vi "Stop Work.vi"(8 "error in (no error)":errorcluster, 9 "Reply":bool=TRUE, 10 "Reply to":refnum<class "Stop Response Msg.lvclass">, 11 "Spectrum Recorder in":refnum<class "Spectrum Recorder too.lvclass">) -> (0 "error out":errorcluster, 3 "Spectrum Recorder out":refnum<class "Spectrum Recorder too.lvclass">)   [LabVIEW 2018, in "Spectrum Recorder too.lvclass"]
uses:
  Spectrum Recorder too.lvclass
  C:/github/LabActor/Template Module/Template Module.lvclass
  Controllers/Process Controller Messages/Stop Response Msg/Stop Response Msg.lvclass
  Template Module/Template Module.lvclass/Template Module.ctl
  Template Module/Read Logger.vi
  Template Module/Write Logger.vi
  Read RP transceiver.vi
  Write RP transceiver.vi
  NHMFL_Core/Libraries/Red Pitaya/RP Core/RP Transceiver/RP Transceiver.lvclass
  Loggers/Logger/Logger.lvclass
  Instrument Actor/Instrument Actor.lvclass
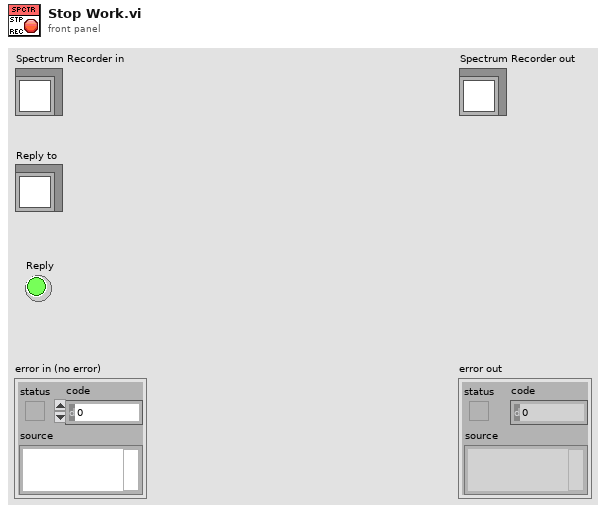
[diagram p1: front panel]
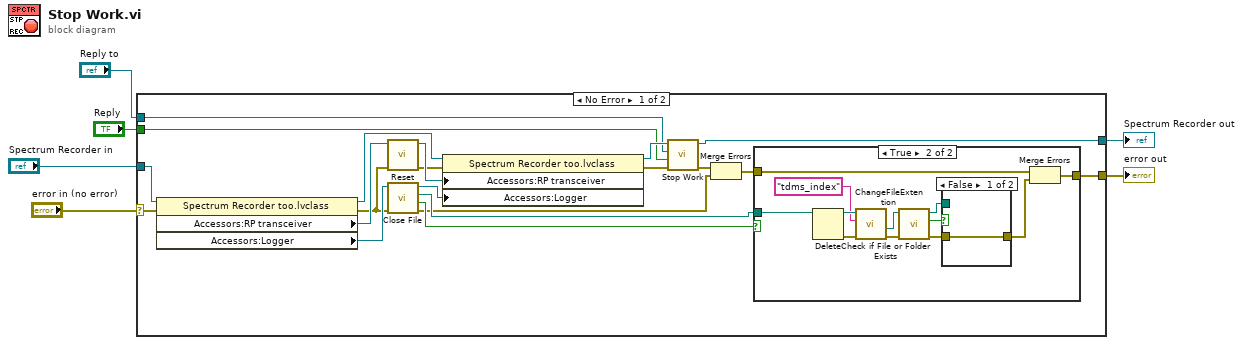
[diagram p0: block diagram]
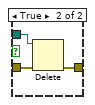
[diagram p3: hidden frame]
diagram:
  n1 = case shown="No Error" "error in (no error)" {
    selector: "error in (no error)" -> [w26 w45]
    tunnel: [w18 w45] -> w5
    tunnel: [w13 w44] -> w3
    tunnel: "Spectrum Recorder in" -> [w23 w44]
    tunnel: "Reply to" -> [w17 _]
    tunnel: "Reply" -> [w16 _]
    frame No Error {
      n2 = property class="Spectrum Recorder too.lvclass"(reference=w23, error in=w26) -> (reference out=w19:refnum<class "Spectrum Recorder too.lvclass">, error out=w10:errorcluster, "Accessors:RP transceiver"=w25:refnum<class "RP Transceiver.lvclass">, "Accessors:Logger"=w11:refnum<class "Logger.lvclass">)
      n3 = call-dynamic "Reset.vi"("error in (no error)"=w10, "RP Instrument in"=w25) -> ("error out"=w20:errorcluster, "RP Instrument out"=w24:refnum<class "RP Transceiver.lvclass">)  [unwired: 8 in]
      n4 = call-dynamic "Close File.vi"("error in (no error)"=w10, "Logger in"=w11) -> ("error out"=w8:errorcluster, "Actually closed"=w14:bool, "File Path"=w12:path, "Logger out"=w7:refnum<class "Logger.lvclass">)  [unwired: 6 in]
      n5 = property class="Spectrum Recorder too.lvclass"(reference=w19, error in=w20, "Accessors:RP transceiver"=w24, "Accessors:Logger"=w7) -> (reference out=w22:refnum<class "Spectrum Recorder too.lvclass">, error out=w21:errorcluster)
      n6 = call-parent "Stop Work.vi"("error in (no error)"=w21, "Reply"=w16, "Reply to"=w17, "Measure Object in"=w22) -> ("error out"=w15:errorcluster, "Measure Object out"=w13:refnum<class "Spectrum Recorder too.lvclass">)  [unwired: 6 in]
      n7 = Merge Errors(w15, w8) -> (w9:errorcluster)
      n8 = case shown="True" w14 {
        tunnel: w9 -> [w27 w34]
        tunnel: [w27 w32] -> w18
        tunnel: w12 -> [_ w28]
        frame False {
        }
        frame True {
          n9 = Delete(path (use dialog)=w28) -> (deleted path=w39:path, error out=w31:errorcluster)  [unwired: 4 in, 1 out]
          n10 = call "ChangeFileExtention.vi"("Error In"=w31, "New extension"="tdms_index" ("New Extention"), "File Path"=w39) -> ("Error Out"=w30:errorcluster, "Path with new extension"=w29:path)  [unwired: 3 in, 4 out]
          n11 = call <vilib>:"Check if File or Folder Exists.vi"("error in (no error)"=w30, "path"=w29) -> ("error out"=w36:errorcluster, "file or folder exists?"=w37:bool, "dup path"=w35:path)  [unwired: 7 in]
          n12 = case shown="False" w37 {
            tunnel: w36 -> [w40 w43]
            tunnel: w35 -> [_ w42]
            tunnel: [w40 w41] -> w33
            frame False {
            }
            frame True {
              n13 = Delete(path (use dialog)=w42, error in=w43) -> (error out=w41:errorcluster)  [unwired: 3 in, 2 out]
            }
          }
          n14 = Merge Errors(w34, w33) -> (w32:errorcluster)
        }
      }
    }
    frame Error {
    }
  }
  "error out" <- w5
  "Spectrum Recorder out" <- w3
